vi "CRYClick Name in Legend.vi"(10 "Mouse Point":T1, 11 "MCListbox Ref In":refnum<vi>) -> (2 "Active Row":i32, 3 "Click State?":bool)   [LabVIEW 2013]
uses:
  <vilib>/Utility/miscctls.llb/LVPositionTypeDef.ctl
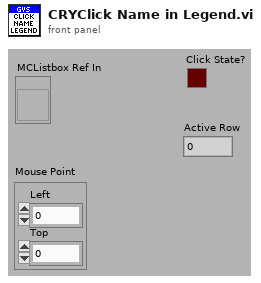
[diagram p1: front panel]
types:
  T1 = typedef "LVPositionTypeDef.ctl" = cluster{"Left":i32, "Top":i32}
  T2 = typedef "LVRowAndColumnTypeDef.ctl" = cluster{"Row":i32, "Column":i32}
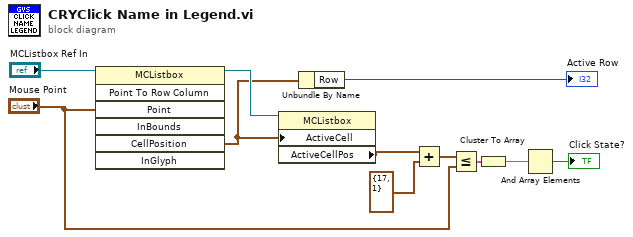
[diagram p0: block diagram]
diagram:
  n1 = invoke on="Invoke Node" class="MCListbox" method="Point To Row Column"(reference="MCListbox Ref In", "Point"="Mouse Point") -> (reference out=w4:refnum<vi>, "CellPosition"=w2:T2)  [unwired: 5 in, 5 out]
  n2 = property on="Property Node" class="MCListbox"(reference=w4, "ActiveCell"=w2) -> ("ActiveCellPos"=w9:T1)  [unwired: 1 in, 2 out]
  n3 = Unbundle By Name(w2) -> ("Row"=→"Active Row":i32)
  n4 = Add(x=w9, y=T1 {"Left"=17, "Top"=1}) -> (x+y=w8:T1)
  n5 = Less Or Equal?(x=w8, y="Mouse Point") -> (x <= y?=w7:cluster{"Left":bool, "Top":bool})
  n6 = Cluster To Array(cluster=w7) -> (array=w5:bool[])
  n7 = And Array Elements(Boolean array=w5) -> (logical AND=→"Click State?":bool)
